vi "START-STOP(SubVI).vi"(8 "error in (no error)":errorcluster, 10 "Enum":enum16{"START DAQ", "STOP DAQ"}(ring), 11 "VISA Refnum in":refnum<visa-resource-name>) -> (0 "error out":errorcluster, 3 "VISA Refnum out":refnum<visa-resource-name>)   [LabVIEW 2014, in "CAP-USB.lvlib"]
doc: "Envia los comandos al CAP-USB para \ncomenzar la adqusicion de datos \no detener el envio."
uses:
  CAP-USB.lvlib
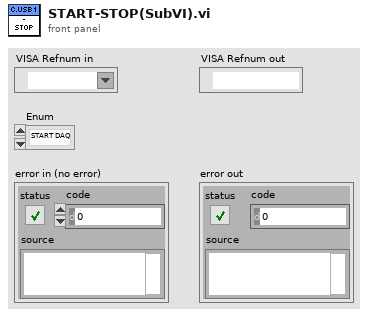
[diagram p1: front panel]
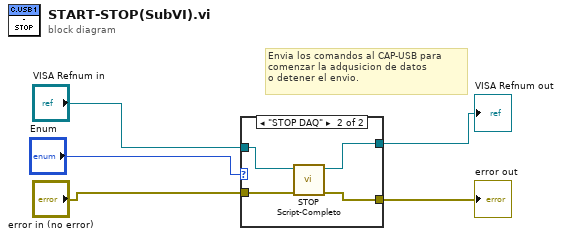
[diagram p0: block diagram]
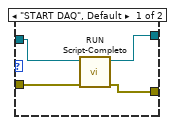
[diagram p2: hidden frame]
diagram:
  # "Envia los comandos al CAP-USB para \ncomenzar la adqusicion de datos \no detener el envio."
  n1 = case shown="\"STOP DAQ\"" "Enum" {
    tunnel: "VISA Refnum in" -> [w9 w13]
    tunnel: "error in (no error)" -> [w8 w12]
    tunnel: [w7 w11] -> w4
    tunnel: [w6 w10] -> w5
    frame "START DAQ", Default {
      n2 = call "RUN Script-Completo.vi"("error in (no error)"=w8, "VISA resource name"=w9) -> ("error out"=w6:errorcluster, "VISA resource name out"=w7:refnum<visa-resource-name>)  [unwired: 8 in]
    }
    frame "STOP DAQ" {
      n3 = call "STOP Script-Completo.vi"("error in (no error)"=w12, "VISA resource name"=w13) -> ("error out"=w10:errorcluster, "VISA resource name out"=w11:refnum<visa-resource-name>)  [unwired: 8 in]
    }
  }
  "error out" <- w5
  "VISA Refnum out" <- w4
